vi "Write User Id.vi"(8 "error in (no error)":errorcluster, 10 "user id":string, 11 "External Calibration Operator in":refnum<class "External Calibration Operator.lvclass">) -> (0 "error out":errorcluster, 3 "External Calibration Operator out":refnum<class "External Calibration Operator.lvclass">)   [LabVIEW 2019, in "External Calibration Operator.lvclass"]
uses:
  External Calibration Operator.lvclass
  External Calibration Operator.lvclass/External Calibration Operator.ctl
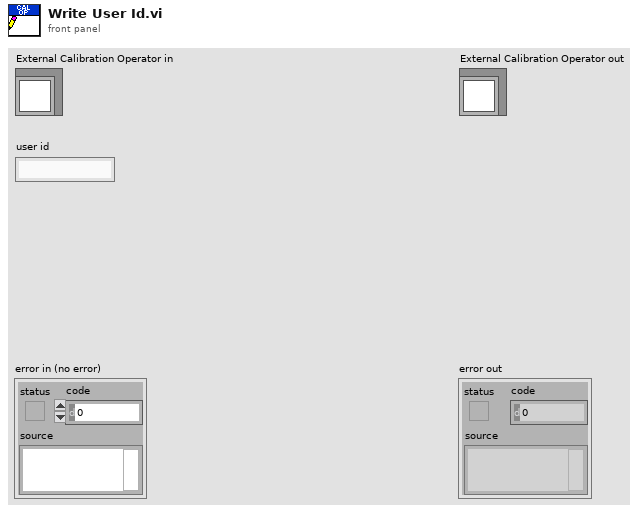
[diagram p1: front panel]
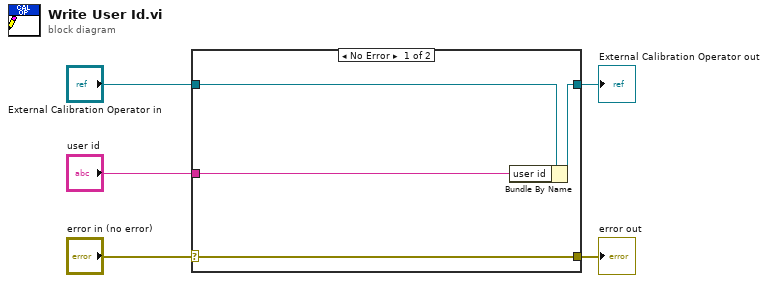
[diagram p0: block diagram]
diagram:
  n1 = case shown="No Error" "error in (no error)" {
    selector: "error in (no error)" -> [w9 w10]
    tunnel: [w9 w10] -> w4
    tunnel: [w7 w11] -> w2
    tunnel: "External Calibration Operator in" -> [w8 w11]
    tunnel: "user id" -> [w6 _]
    frame No Error {
      n2 = Bundle By Name(cluster=w8, "user id"=w6) -> (w7:refnum<class "External Calibration Operator.lvclass">)
    }
    frame Error {
    }
  }
  "error out" <- w4
  "External Calibration Operator out" <- w2
